vi "Configure Baud Rate.vi"(8 "error in (no error)":errorcluster, 10 "baud rate":u32(ring)=115200 items=["9600"=9600, "19200"=19200, "38400"=38400, "57600"=57600, "115200"=115200], 11 "VGC in":refnum<class "PL Inficon VGC.lvclass">) -> (0 "error out":errorcluster, 2 "baud rate":u32(ring)=115200 items=["9600"=9600, "19200"=19200, "38400"=38400, "57600"=57600, "115200"=115200], 3 "VGC out":refnum<class "PL Inficon VGC.lvclass">)   [LabVIEW 2015, in "PL Inficon VGC.lvclass"]
doc: "Configures baud rate."
uses:
  PL Inficon VGC.lvclass
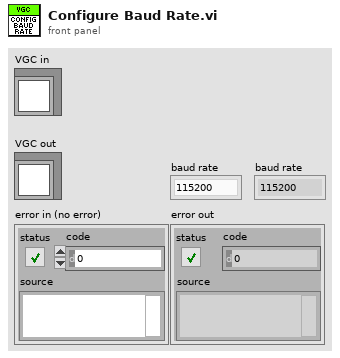
[diagram p1: front panel]
types:
  T1 = typedef "LVStringsAndValuesArrayTypeDef_U32.ctl" = cluster{"String":string, "Value":u32}[]
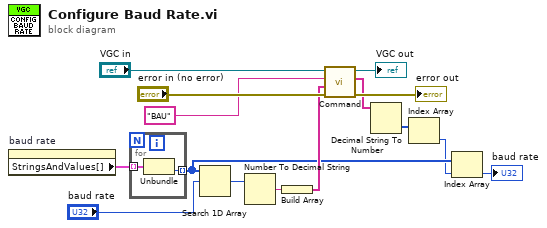
[diagram p0: block diagram]
diagram:
  n1 = property on="baud rate" class="Ring (strict)"() -> ("StringsAndValues[]"=w6:T1)  [unwired: 2 in, 2 out]
  n2 = for {
    tunnel: w6 -> [w17] mode=indexing
    tunnel: [w16] -> w3 mode=indexing
    n3 = Unbundle(w17) -> ("Value"=w16:u32)  [unwired: 1 out]
  }
  n4 = Search 1D Array(1D array=w3, element="baud rate") -> (index of element=w4:i32)  [unwired: 1 in]
  n5 = Number To Decimal String(number=w4) -> (decimal integer string=w11:string)  [unwired: 1 in]
  n6 = Build Array(w11) -> (w10:string[])
  n7 = call "Command.vi"("error in (no error)"="error in (no error)", "parameters"=w10, "command"="BAU" ("format string"), "VGC in"="VGC in") -> ("error out"=→"error out":errorcluster, "response data"=w8:string[], "VGC out"=→"VGC out":refnum<class "PL Inficon VGC.lvclass">)  [unwired: 5 in]
  n8 = Decimal String To Number(string=w8) -> (number=w9:i32[])  [unwired: 2 in, 1 out]
  n9 = Index Array(array=w9) -> (element=w2:i32)  [unwired: 1 in]
  n10 = Index Array(array=w3, index=w2) -> (element=→"baud rate":u32)
